vi "Is Safe to Destroy Refnums.vi"(8 "error in":errorcluster, 10 "empty":bool, 11 "Module Admin":refnum<class "Delacor_lib_QMH_Cloneable Module Admin.lvclass">) -> (0 "error out":errorcluster, 3 "Destroy Broadcast & Request Event Refs?":bool)   [LabVIEW 2025, in "Test Unit.lvlib"]
doc: "If this cloneable module instance was the first one that was launched, wait until all other instances are closed, then indicate that it is safe to destroy the event references.\n_____\nBased on DQMH Project Template 7.0.1.1316."
uses:
  Test Unit.lvlib
  <vilib>/Delacor/Delacor QMH/Libraries/Cloneable Module Admin_class/Delacor_lib_QMH_Cloneable Module Admin.lvclass
  <vilib>/Delacor/Delacor QMH/Libraries/Cloneable Module Admin_class/Delacor_lib_QMH_Cloneable Module Admin.lvclass/Delacor_lib_QMH_Cloneable Module Admin.ctl
  <vilib>/Delacor/Delacor QMH/Libraries/Cloneable Module Admin_class/Delacor_lib_QMH_Get First.vi
  Clone Registration/Clone Registration.lvlib
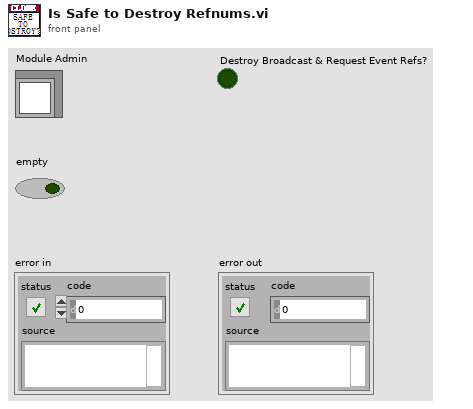
[diagram p1: front panel]
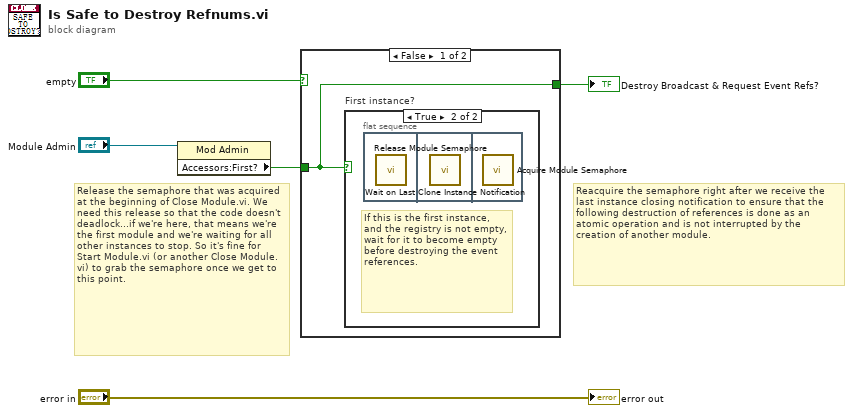
[diagram p0: block diagram]
diagram:
  # "Reacquire the semaphore right after we receive the last instance closing notification to ensure that the following destruction of references is done as an atomic operation and is not interrupted by the creation of another module."
  # "Release the semaphore that was acquired at the beginning of Close Module.vi. We need this release so that the code doesn't deadlock...if we're here, that means we're the first module and we're waiting for all other instances to stop. So it's fine for Start Module.vi (or another Close Module.vi) to grab the semaphore once we get to this point."
  n1 = property class="Mod Admin"(reference="Module Admin") -> ("Accessors:First?"=w2:bool)  [unwired: 1 in, 2 out]
  n2 = case shown="False" "empty" {
    tunnel: w2 -> [w6 w7]
    tunnel: [w6 w7] -> w1
    frame False {
      n3 = case "First instance?" shown="True" w6 {
        frame False {
          # "This is not the first instance, so don't try to destroy the event references."
        }
        frame True {
          # "If this is the first instance, and the registry is not empty, wait for it to become empty before destroying the event references."
          n4 = flat-sequence {
            frame #0 {
              n5 = call "Release Module Semaphore.vi"() -> ()  [unwired: 11 in, 1 out]
            }
            frame #1 {
              n6 = call "Wait on Last Clone Instance Notification.vi"() -> ()  [unwired: 12 in]
            }
            frame #2 {
              n7 = call "Acquire Module Semaphore.vi"() -> ()  [unwired: 11 in, 1 out]
            }
          }
        }
      }
    }
    frame True {
      # "The registry is empty. If this was the first module, it is ok to destroy the event references."
    }
  }
  "Destroy Broadcast & Request Event Refs?" <- w1
  "error out" <- "error in"
